vi "KeyEvent.vi"(8 "error in (no error)":errorcluster, 10 "Keys Pressed":T1(array[ring]), 11 "Menu in":refnum<class "Menu.lvclass">) -> (0 "error out":errorcluster, 3 "Menu out":refnum<class "Menu.lvclass">)   [LabVIEW 2021, in "Menu.lvlib" / "Menu.lvclass"]
uses:
  Menu.lvclass
  <vilib>/Utility/miscctls.llb/LVMenuShortCut.ctl
  MenuSelection.ctl
  <vilib>/event_ctls.llb/usereventprio.ctl
  d9c172c7-d3bb-4bd5-a19d-c419eb0dd62c.vi
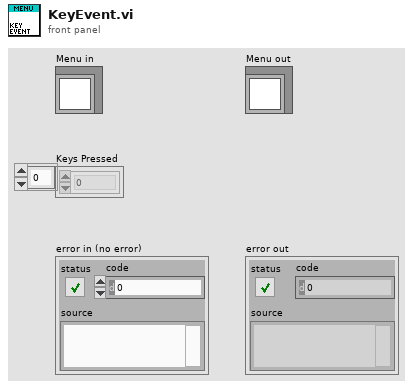
[diagram p1: front panel]
types:
  T1 = enum16{"0", "1", "2", "3", "4", "5", "6", "7", "8", "9", "A", "B", "C", "D", "E", "F", "G", "H", "I", "J", "K", "L", "M", "N", "O", "P", "Q", "R", "S", "T", "U", "V", "W", "X", "Y", "Z", "F1", "F2", "F3", "F4", "F5", "F6", "F7", "F8", "F9", "F10", "F11", "F12", "F13", "F14", "F15", "ADD", "BACK", "BACKSLASH", "CAPITAL", "COMMA", "DECIMAL", "DELETE", "DIVIDE", "DOWN", "END", "EQUALS", "ESCAPE", "GRAVE (`)", "HOME", "INSERT", "LBRACKET", "LCONTROL", "LEFT", "L ALT", "LSHIFT", "LWIN", "MINUS", "MULTIPLY", "NEXT", "NUMLOCK", "NUMPAD_0", "NUMPAD_1", "NUMPAD_2", "NUMPAD_3", "NUMPAD_4", "NUMPAD_5", "NUMPAD_6", "NUMPAD_7", "NUMPAD_8", "NUMPAD_9", "PAUSE", "PERIOD", "PRIOR (PG UP)", "RBRACKET", "RCONTROL", "RETURN", "RIGHT", "R ALT", "RSHIFT", "RWIN", "SCROLL", "SEMICOLON", "SLASH", "SPACE", "SUBTRACT", "TAB", "UP", "ENTER (num pad)", "' (quote)"}[]
  T2 = enum16{"LSHIFT", "RSHIFT", "LCONTROL", "RCONTROL", "OtherChar"}
  T3 = typedef "LVMenuShortCut.ctl" = cluster{"Include Shift Key?":bool, "Include Ctrl Key?":bool, "Shortcut Key":string}
  T4 = enum16{"0", "1", "2", "3", "4", "5", "6", "7", "8", "9", "A", "B", "C", "D", "E", "F", "G", "H", "I", "J", "K", "L", "M", "N", "O", "P", "Q", "R", "S", "T", "U", "V", "W", "X", "Y", "Z", "F1", "F2", "F3", "F4", "F5", "F6", "F7", "F8", "F9", "F10", "F11", "F12", "F13", "F14", "F15", "ADD", "BACK", "BACKSLASH", "CAPITAL", "COMMA", "DECIMAL", "DELETE", "DIVIDE", "DOWN", "END", "EQUALS", "ESCAPE", "GRAVE (`)", "HOME", "INSERT", "LBRACKET", "LCONTROL", "LEFT", "L ALT", "LSHIFT", "LWIN", "MINUS", "MULTIPLY", "NEXT", "NUMLOCK", "NUMPAD_0", "NUMPAD_1", "NUMPAD_2", "NUMPAD_3", "NUMPAD_4", "NUMPAD_5", "NUMPAD_6", "NUMPAD_7", "NUMPAD_8", "NUMPAD_9", "PAUSE", "PERIOD", "PRIOR (PG UP)", "RBRACKET", "RCONTROL", "RETURN", "RIGHT", "R ALT", "RSHIFT", "RWIN", "SCROLL", "SEMICOLON", "SLASH", "SPACE", "SUBTRACT", "TAB", "UP", "ENTER (num pad)", "' (quote)"}
  T5 = typedef "usereventprio.ctl" = enum32{"high priority", "normal priority"}
  T6 = typedef "Menu.lvlib/Menu.lvclass/MenuSelection.ctl" = cluster{"ItemTag":string, "ItemPath":string}
  T7 = enum16{"LSHIFT", "RSHIFT", "LCONTROL", "RCONTROL", "OtherChar"}[]
  T8 = typedef "Menu.lvlib/Menu.lvclass/Data.ctl" = cluster{"MenuMap":map{string, T9}, "PictRef":refnum<vi>, "MenuSelectionEvent":refnum<user-event>, "TopMenuSpacing":i32, "MenuSpacing":i32, "CloseEvent":refnum<user-event>, "TR_ManageMenuRef":refnum<vi>, "MenuColors":T10, "RTMPath":path, "RTMVIReference":refnum<vi>, "RTMMenuReference":refnum<k9>, "CtlRef":refnum<vi>, "User-Specified Font":refnum<class "Font.lvclass">, "Desired Font":enum16{"User-specified Font", "Application Font", "System Font", "Dialog Font"}, "SubMenuIcon":T11, "SubMenuIconClosed":refnum<class "Picture2D.lvclass">, "SubMenuIconOpened":refnum<class "Picture2D.lvclass">}
  T9 = typedef "Menu.lvlib/Menu.lvclass/MenuItems.ctl" = cluster{"Item Name":string, "Short Cut":T3, "Checked":bool, "Enable":bool, "After item":string, "Item Tags":string[], "Item Names":string[], "Picture":refnum<class "Image.lvclass">, "Hilite Picture":refnum<class "Image.lvclass">, "Displayed":bool}
  T10 = typedef "Menu.lvlib/Menu.lvclass/MenuColors.ctl" = cluster{"Text":refnum<class "Color.lvclass">, "HiliteText":refnum<class "Color.lvclass">, "Background":refnum<class "Color.lvclass">, "BorderColor":refnum<class "Color.lvclass">, "Hilite":refnum<class "Color.lvclass">}
  T11 = typedef "Menu.lvlib/Menu.lvclass/SubMenuIcon.ctl" = enum16{"LabVIEW", "Windows", "Custom"}
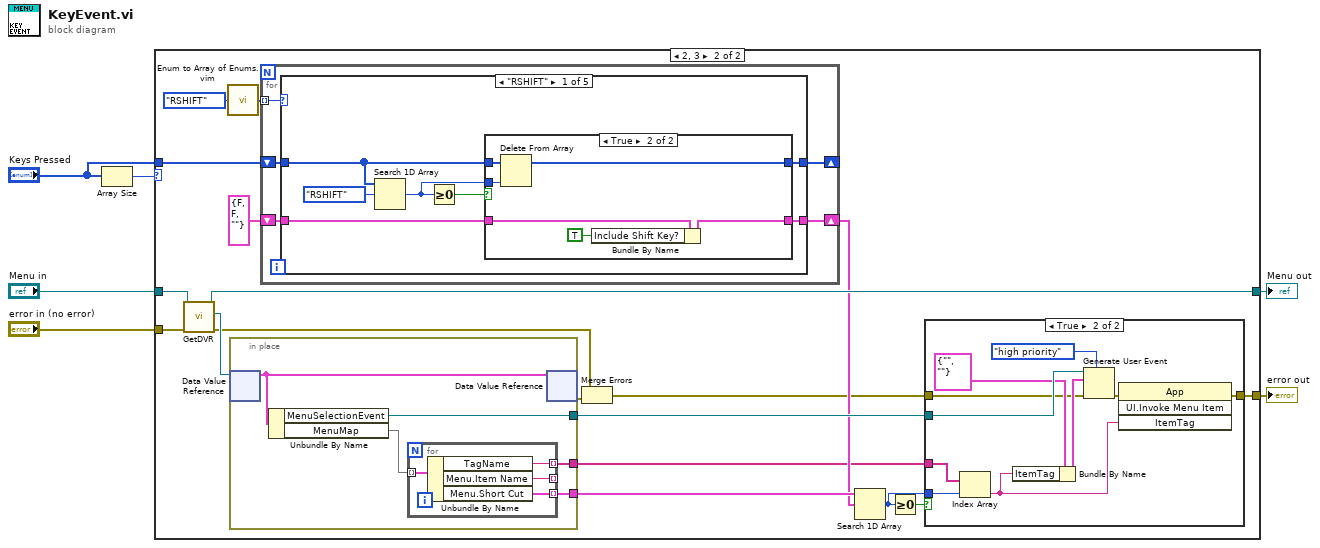
[diagram p0: block diagram]
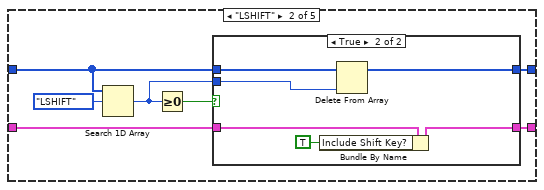
[diagram p4: hidden frame]
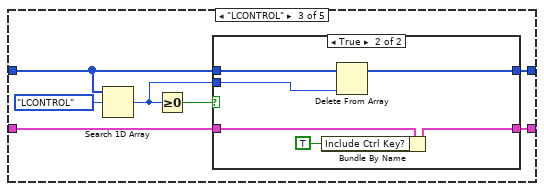
[diagram p6: hidden frame]
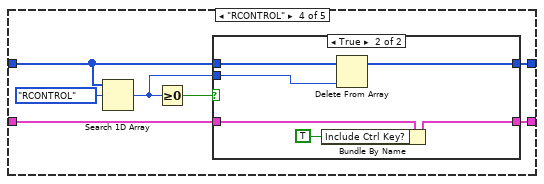
[diagram p8: hidden frame]
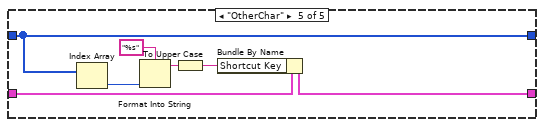
[diagram p10: hidden frame]
diagram:
  n1 = Array Size(array="Keys Pressed") -> (size(s)=w3:i32)
  n2 = case shown="2, 3" w3 {
    tunnel: "Menu in" -> [w7 w26]
    tunnel: [w8 w11] -> w6
    tunnel: "error in (no error)" -> [w8 w10]
    tunnel: "Keys Pressed" -> [_ w20]
    tunnel: [w7 w19] -> w1
    frame ..1, 4.. {
    }
    frame 2, 3 {
      n3 = call "GetDVR.vi"("error in (no error)"=w10, "Menu in"=w26) -> ("error out"=w9:errorcluster, "DVR"=w25:refnum<data-value>, "Menu out"=w19:refnum<class "Menu.lvclass">)  [unwired: 7 in]
      n4 = call "Enum to Array of Enums.vim"("enum"=T2."RSHIFT") -> ("array of enums"=w22:T7)
      n5 = in-place {
        in-place-border: [w99] -> w24
        in-place-border: [w101] -> w17
        in-place-border: [w100] -> w14
        n6 = in-place-dvr #1(w25) -> (w102:T8)  [unwired: 1 out]
        n7 = Unbundle By Name(w102) -> ("MenuSelectionEvent"=w99:refnum<user-event>, "MenuMap"=w103:map{string, T9})
        n8 = for {
          tunnel: w103 -> [w107] mode=indexing
          tunnel: [w106] -> w100 mode=indexing
          tunnel: [w105] -> _ mode=indexing
          tunnel: [w104] -> w101 mode=indexing
          n9 = Unbundle By Name(w107) -> ("TagName"=w106:string, "Menu.Item Name"=w105:string, "Menu.Short Cut"=w104:T3)
        }
        n10 = in-place-dvr #1(w102) -> (w21:errorcluster)  [unwired: 1 out]
      }
      n11 = for {
        shift-right: [w28] -> w16
        shift-left: T3 {"Include Shift Key?"=FALSE, "Include Ctrl Key?"=FALSE, "Shortcut Key"=""} ("Short Cut") -> [w30]
        tunnel: w22 -> [w27] mode=indexing
        shift-right: [w29] -> _
        shift-left: w20 -> [w31]
        n12 = case shown="\"RSHIFT\"" w27 {
          tunnel: w31 -> [w37 w52 w67 w82 w92]
          tunnel: w30 -> [w36 w51 w66 w81 w98]
          tunnel: [w35 w50 w65 w80 w92] -> w29
          tunnel: [w34 w49 w64 w79 w97] -> w28
          frame "RSHIFT" {
            n13 = Search 1D Array(1D array=w37, element=T4."RSHIFT") -> (index of element=w33:i32)  [unwired: 1 in]
            n14 = Greater Or Equal To 0?(x=w33) -> (x >= 0?=w32:bool)
            n15 = case shown="True" w32 {
              tunnel: w37 -> [w39 w42]
              tunnel: w36 -> [w40 w46]
              tunnel: [w40 w45] -> w34
              tunnel: [w39 w43] -> w35
              tunnel: w33 -> [_ w41]
              frame False {
              }
              frame True {
                n16 = Delete From Array(array=w42, index=w41) -> (array with subset deleted=w43:T1)  [unwired: 1 in, 1 out]
                n17 = Bundle By Name(cluster=w46, "Include Shift Key?"=TRUE) -> (w45:T3)
              }
            }
          }
          frame "LSHIFT" {
            n18 = Search 1D Array(1D array=w52, element=T4."LSHIFT") -> (index of element=w48:i32)  [unwired: 1 in]
            n19 = Greater Or Equal To 0?(x=w48) -> (x >= 0?=w47:bool)
            n20 = case shown="True" w47 {
              tunnel: w52 -> [w54 w57]
              tunnel: w51 -> [w55 w61]
              tunnel: [w55 w60] -> w49
              tunnel: [w54 w58] -> w50
              tunnel: w48 -> [_ w56]
              frame False {
              }
              frame True {
                n21 = Bundle By Name(cluster=w61, "Include Shift Key?"=TRUE) -> (w60:T3)
                n22 = Delete From Array(array=w57, index=w56) -> (array with subset deleted=w58:T1)  [unwired: 1 in, 1 out]
              }
            }
          }
          frame "LCONTROL" {
            n23 = Search 1D Array(1D array=w67, element=T4."LCONTROL") -> (index of element=w63:i32)  [unwired: 1 in]
            n24 = Greater Or Equal To 0?(x=w63) -> (x >= 0?=w62:bool)
            n25 = case shown="True" w62 {
              tunnel: w67 -> [w69 w72]
              tunnel: w66 -> [w70 w76]
              tunnel: [w70 w75] -> w64
              tunnel: [w69 w73] -> w65
              tunnel: w63 -> [_ w71]
              frame False {
              }
              frame True {
                n26 = Bundle By Name(cluster=w76, "Include Ctrl Key?"=TRUE ("Include Shift Key?")) -> (w75:T3)
                n27 = Delete From Array(array=w72, index=w71) -> (array with subset deleted=w73:T1)  [unwired: 1 in, 1 out]
              }
            }
          }
          frame "RCONTROL" {
            n28 = Search 1D Array(1D array=w82, element=T4."RCONTROL") -> (index of element=w78:i32)  [unwired: 1 in]
            n29 = Greater Or Equal To 0?(x=w78) -> (x >= 0?=w77:bool)
            n30 = case shown="True" w77 {
              tunnel: w82 -> [w84 w87]
              tunnel: w81 -> [w85 w91]
              tunnel: [w85 w90] -> w79
              tunnel: [w84 w88] -> w80
              tunnel: w78 -> [_ w86]
              frame False {
              }
              frame True {
                n31 = Bundle By Name(cluster=w91, "Include Ctrl Key?"=TRUE ("Include Shift Key?")) -> (w90:T3)
                n32 = Delete From Array(array=w87, index=w86) -> (array with subset deleted=w88:T1)  [unwired: 1 in, 1 out]
              }
            }
          }
          frame "OtherChar" {
            n33 = Index Array(array=w92) -> (element=w96:T4)  [unwired: 1 in]
            n34 = Format Into String(format string="%s", w96) -> (resulting string=w94:string)  [unwired: 2 in, 1 out]
            n35 = To Upper Case(1:w94) -> (0:w93:string)
            n36 = Bundle By Name(cluster=w98, "Shortcut Key"=w93) -> (w97:T3)
          }
        }
      }
      n37 = Merge Errors(w9, w21) -> (w12:errorcluster)
      n38 = Search 1D Array(1D array=w17, element=w16) -> (index of element=w13:i32)  [unwired: 1 in]
      n39 = Greater Or Equal To 0?(x=w13) -> (x >= 0?=w15:bool)
      n40 = case shown="True" w15 {
        tunnel: w24 -> [_ w118]
        tunnel: w14 -> [_ w114]
        tunnel: w13 -> [_ w113]
        tunnel: w12 -> [w108 w110]
        tunnel: [w108 w109] -> w11
        frame False {
        }
        frame True {
          n41 = Index Array(array=w114, index=w113) -> (element=w112:string)
          n42 = Bundle By Name(cluster=T6 {"ItemTag"="", "ItemPath"=""} ("event data"), "ItemTag"=w112) -> (w116:T6)
          n43 = Generate User Event(priority (normal)=usereventprio."high priority", user event=w118, event data cluster=w116, error in=w110) -> (error out=w111:errorcluster)  [unwired: 1 out]
          n44 = invoke class="App" method="UI.Invoke Menu Item"(error in=w111, "ItemTag"=w112) -> (error out=w109:errorcluster)  [unwired: 2 in, 3 out]
        }
      }
    }
  }
  "error out" <- w6
  "Menu out" <- w1
